vi "THRASH Algorithm Final.vi"() -> ()   [LabVIEW 2021]
panel:
  in  "Signal to Noise Threshold":dbl
  in  "THRASH m/z Windows":dbl=3.0
  in  "Average - End Spectrum":dbl=1.0 min=1.0
  in  "Average - Starting Spectrum":dbl min=0.0
  out "Errors":errorcluster
  out "Average Mass Spectrum":T1(graph)
  out "Total Ion Chromatogram":dbl[](graph)
  in  "File Path":path
  # "Things software could do with:\n\nAbility to remove individual points and update accordingly"
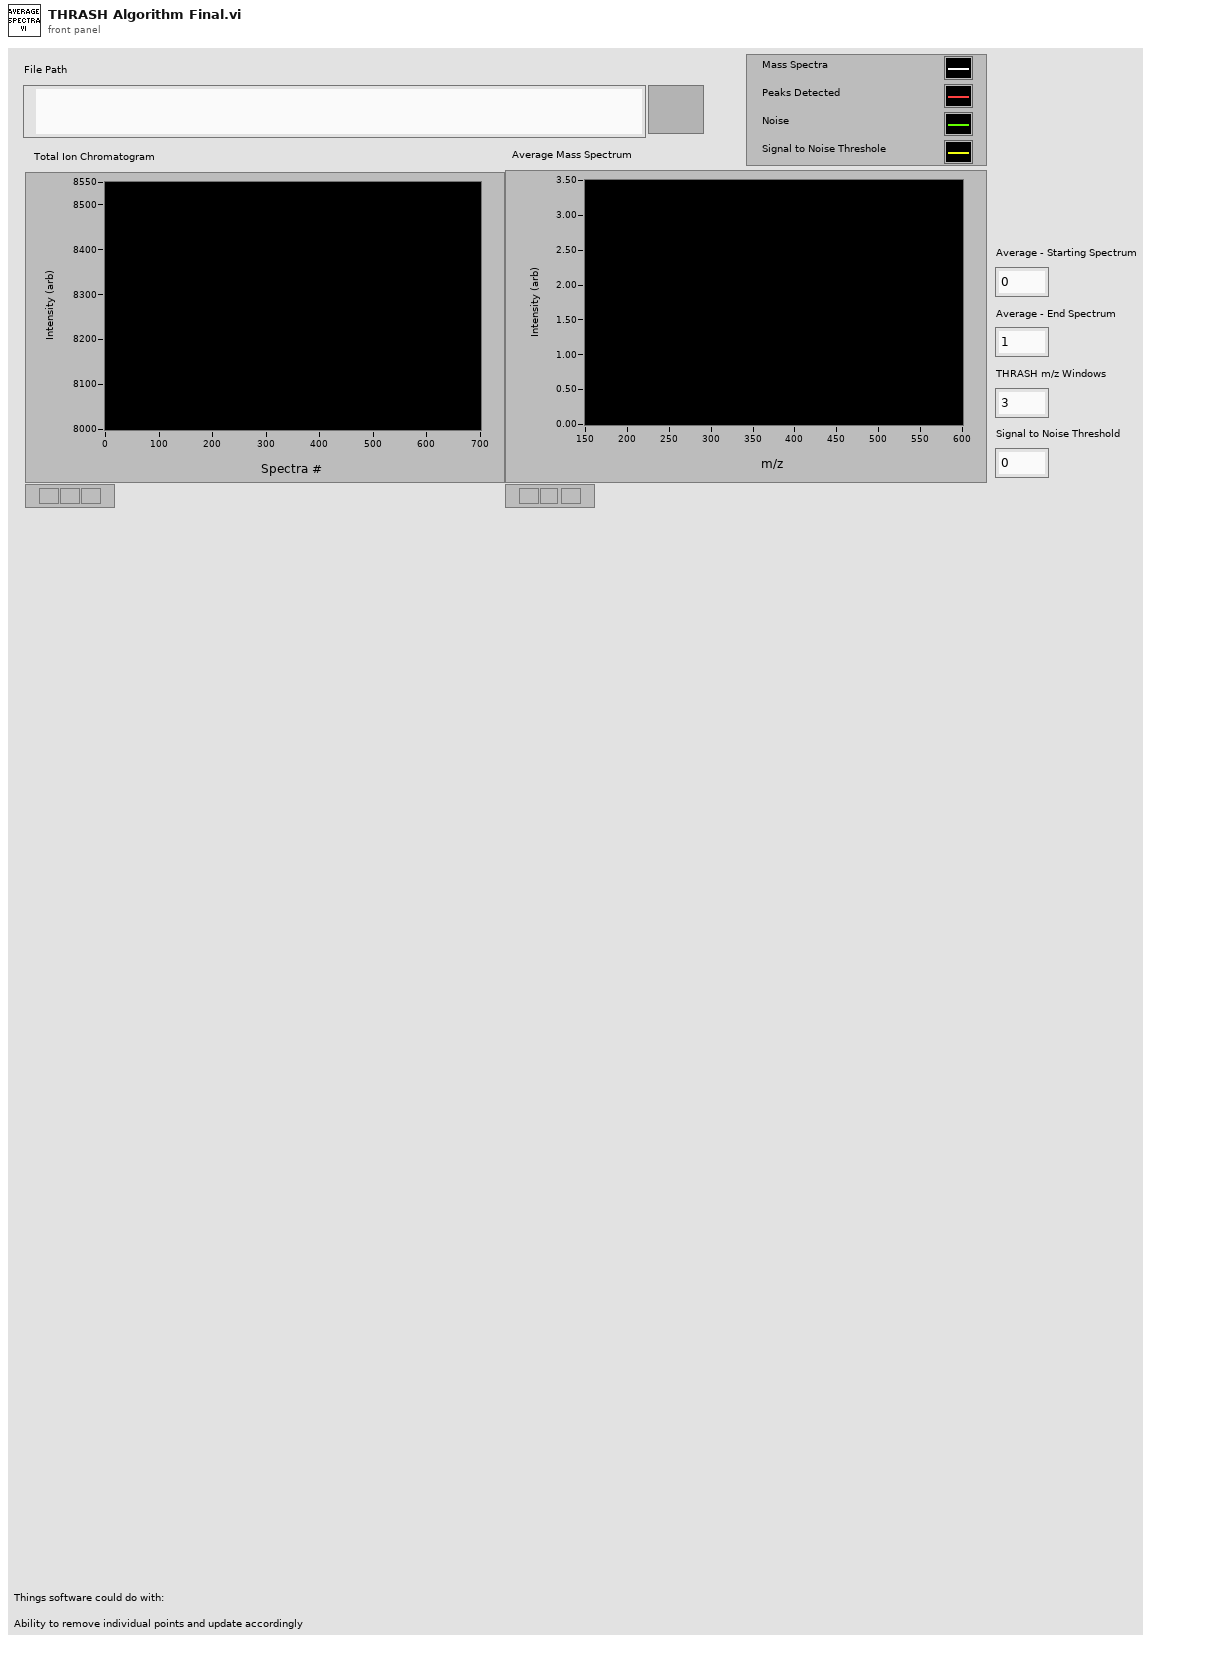
[diagram p1: front panel]
types:
  T1 = cluster{dbl[], "Averaged Intensity Values":dbl[]}[]
  T2 = cluster{dbl[], "Averaged Intensity Values":dbl[]}
  T3 = cluster{"Peak m/z":dbl[], "Peak Intensities":dbl[]}
  T4 = cluster{"Peak m/z":dbl[], "Peak Intensities":dbl[]}[]
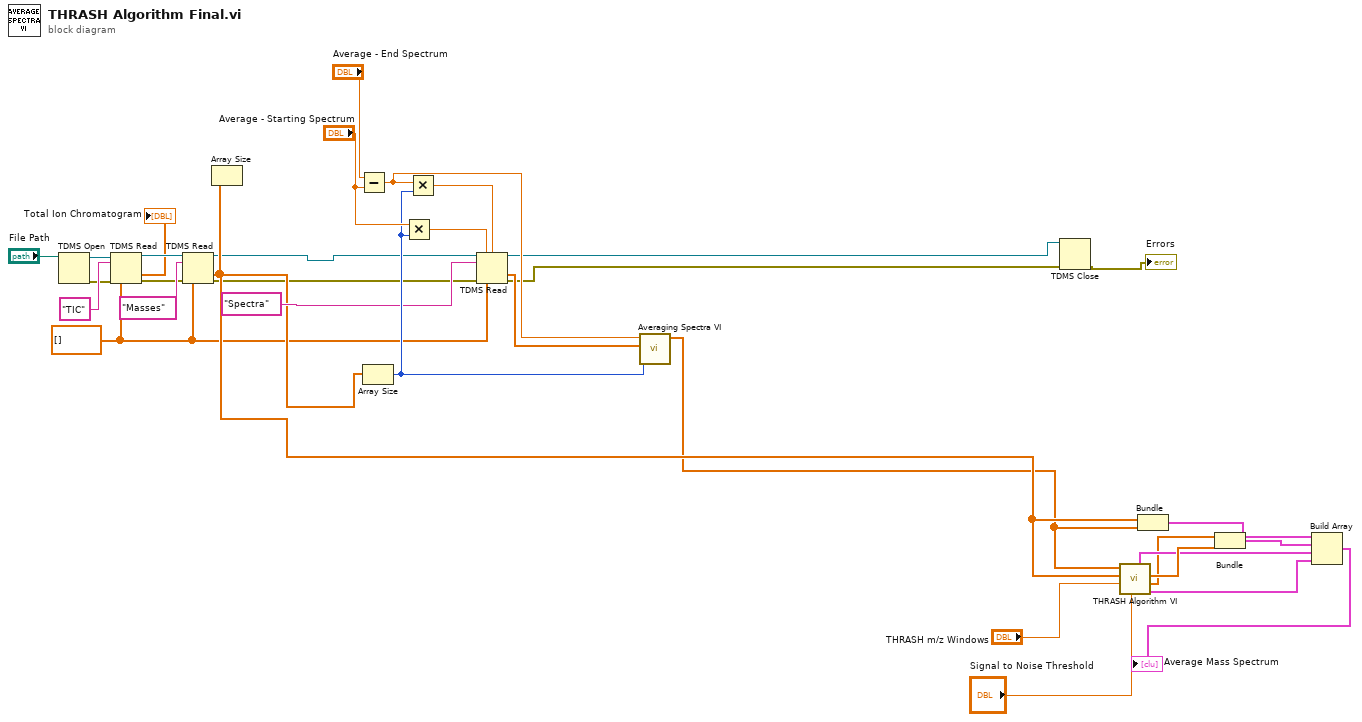
[diagram p0: block diagram]
diagram:
  w2 = dbl[] []
  n1 = TDMS Open(11:"File Path") -> (0:w21:errorcluster, 3:w22:refnum<k34>)  [unwired: 6 in]
  n2 = TDMS Read(0:w22, 5:"TIC" ("group name in"), 11:w21, 12:w2) -> (4:w31:refnum<k34>, 10:→"Total Ion Chromatogram":dbl[], 15:w30:errorcluster)  [unwired: 4 in, 3 out]
  n3 = TDMS Read(0:w31, 5:"Masses" ("group name in"), 11:w30, 12:w2) -> (4:w3:refnum<k34>, 10:w11:dbl[], 15:w1:errorcluster)  [unwired: 4 in, 3 out]
  n4 = Array Size(array=w11) -> ()  [unwired: 1 out]
  n5 = Subtract(x="Average - End Spectrum", y="Average - Starting Spectrum") -> (x-y=w20:dbl)
  n6 = Array Size(array=w11) -> (size(s)=w23:i32)
  n7 = Multiply(x="Average - Starting Spectrum", y=w23) -> (x*y=w25:dbl)
  n8 = Multiply(x=w20, y=w23) -> (x*y=w27:dbl)
  n9 = TDMS Read(0:w3, 1:w25, 2:w27, 5:"Spectra" ("group name in"), 11:w1, 12:w2) -> (4:w6:refnum<k34>, 10:w24:dbl[], 15:w5:errorcluster)  [unwired: 2 in, 3 out]
  n10 = call "Averaging Spectra VI.vi"("Number of Masses"=w23, "Spectra In"=w24, "Spectra Range to be Averaged"=w20) -> ("Averaged Intensity Values"=w7:dbl[])  [unwired: 8 in]
  n11 = TDMS Close(8:w5, 11:w6) -> (0:→"Errors":errorcluster)  [unwired: 1 out]
  n12 = call "THRASH Algorithm VI.vi"("Signal to Noise"="Signal to Noise Threshold", "THRASH Algorithm m/z Windows"="THRASH m/z Windows", "m/z"=w11, "Averaged Intensity Values"=w7) -> ("SNR Threshold"=w12:cluster{dbl[], dbl[]}, "Peak m/z"=w8:dbl[], "Peak Intensities"=w15:dbl[], "Noise Levels"=w13:cluster{dbl[], dbl[]})  [unwired: 3 in, 1 out]
  n13 = Bundle(w11, "Averaged Intensity Values"=w7) -> (w17:T2)  [unwired: 1 in]
  n14 = Bundle("Peak m/z"=w8, "Peak Intensities"=w15) -> (w14:T3)  [unwired: 1 in]
  n15 = Build Array(w17, w14, w13, w12) -> (→"Average Mass Spectrum":T4)
